vi "Write Waveform data.vi"(8 "error in (no error)":errorcluster, 10 "Waveform data":waveform(dbl), 11 "1D wfm (DBL) Result in":refnum<class "1D wfm (DBL) Result.lvclass">) -> (0 "error out":errorcluster, 3 "1D wfm (DBL) Result out":refnum<class "1D wfm (DBL) Result.lvclass">)   [LabVIEW 2015, in "1D wfm (DBL) Result.lvclass"]
uses:
  1D wfm (DBL) Result.lvclass
  1D wfm (DBL) Result.lvclass/1D wfm (DBL) Result.ctl
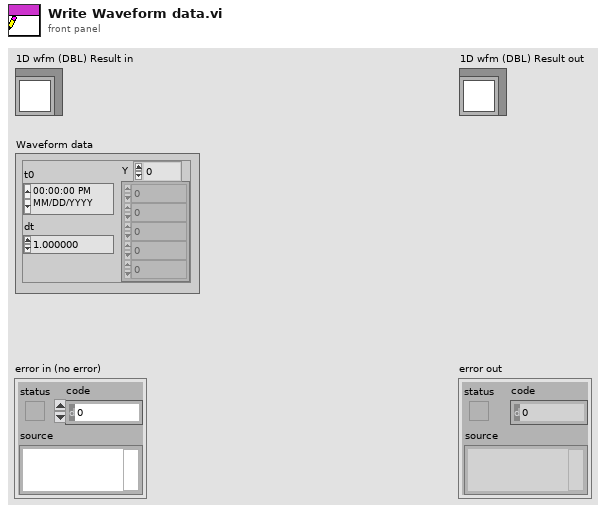
[diagram p1: front panel]
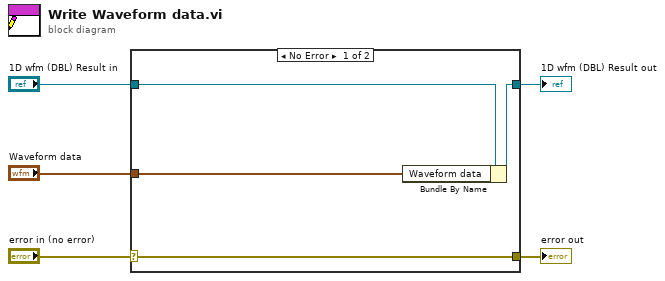
[diagram p0: block diagram]
diagram:
  n1 = case shown="No Error" "error in (no error)" {
    selector: "error in (no error)" -> [w9 w10]
    tunnel: [w9 w10] -> w4
    tunnel: [w7 w11] -> w2
    tunnel: "1D wfm (DBL) Result in" -> [w8 w11]
    tunnel: "Waveform data" -> [w6 _]
    frame No Error {
      n2 = Bundle By Name(cluster=w8, "Waveform data"=w6) -> (w7:refnum<class "1D wfm (DBL) Result.lvclass">)
    }
    frame Error {
    }
  }
  "error out" <- w4
  "1D wfm (DBL) Result out" <- w2
